vi "1.vi"(8 "error in (no error)":errorcluster, 11 "r":dbl) -> (0 "error out":errorcluster, 3 "A":dbl)   [LabVIEW 2020]
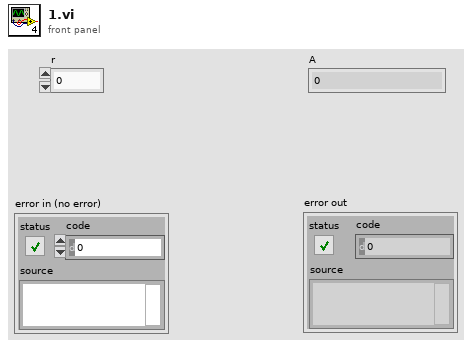
[diagram p1: front panel]
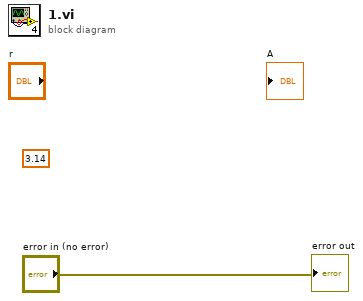
[diagram p0: block diagram]
diagram:
  (unwired) 3.14
  "error out" <- "error in (no error)"
